vi "Process.vi"(11 "jettl Actor in":refnum<class "jettl Actor.lvclass">) -> (3 "jettl Actor out":refnum<class "jettl Actor.lvclass">)   [LabVIEW 2021, in "jettl.lvlib" / "Temporary Actor.lvlib" / "jettl Actor.lvclass"]
uses:
  jettl Actor.lvclass
  jettl Actor.lvclass/jettl Actor.ctl
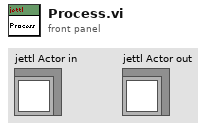
[diagram p1: front panel]
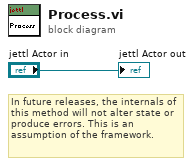
[diagram p0: block diagram]
diagram:
  # "In future releases, the internals of this method will not alter state or produce errors. This is an assumption of the framework."
  "jettl Actor out" <- "jettl Actor in"
